vi "ExportMeasuresToHTML.vi"(8 "error in (no error)":errorcluster, 11 "Table in":refnum<vi>) -> (0 "error out":errorcluster)   [LabVIEW 2013]
uses:
  GlobalVariables/UserInfos.vi
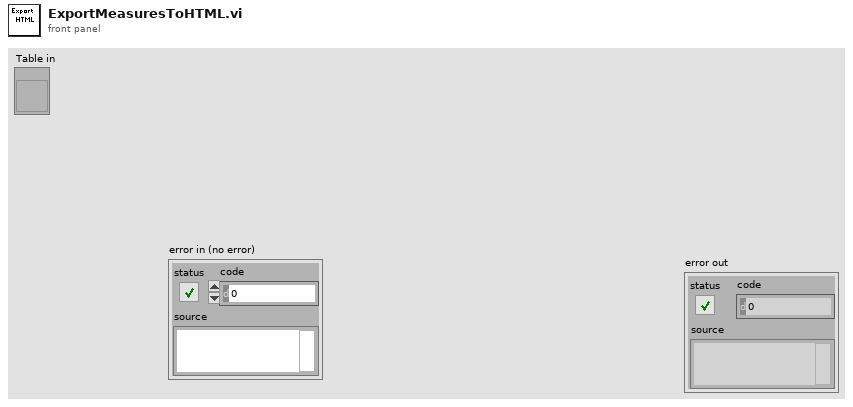
[diagram p1: front panel]
types:
  T1 = enum16{"open", "replace", "create", "open or create", "replace or create", "replace or create with confirmation"}
  T2 = cluster{"location":string, "Field":string, "Company":string, "Lab":string, "Operator":string, "Well":string, "Lat/Long":string, "Formation":string, "Country":string, "Client":string}
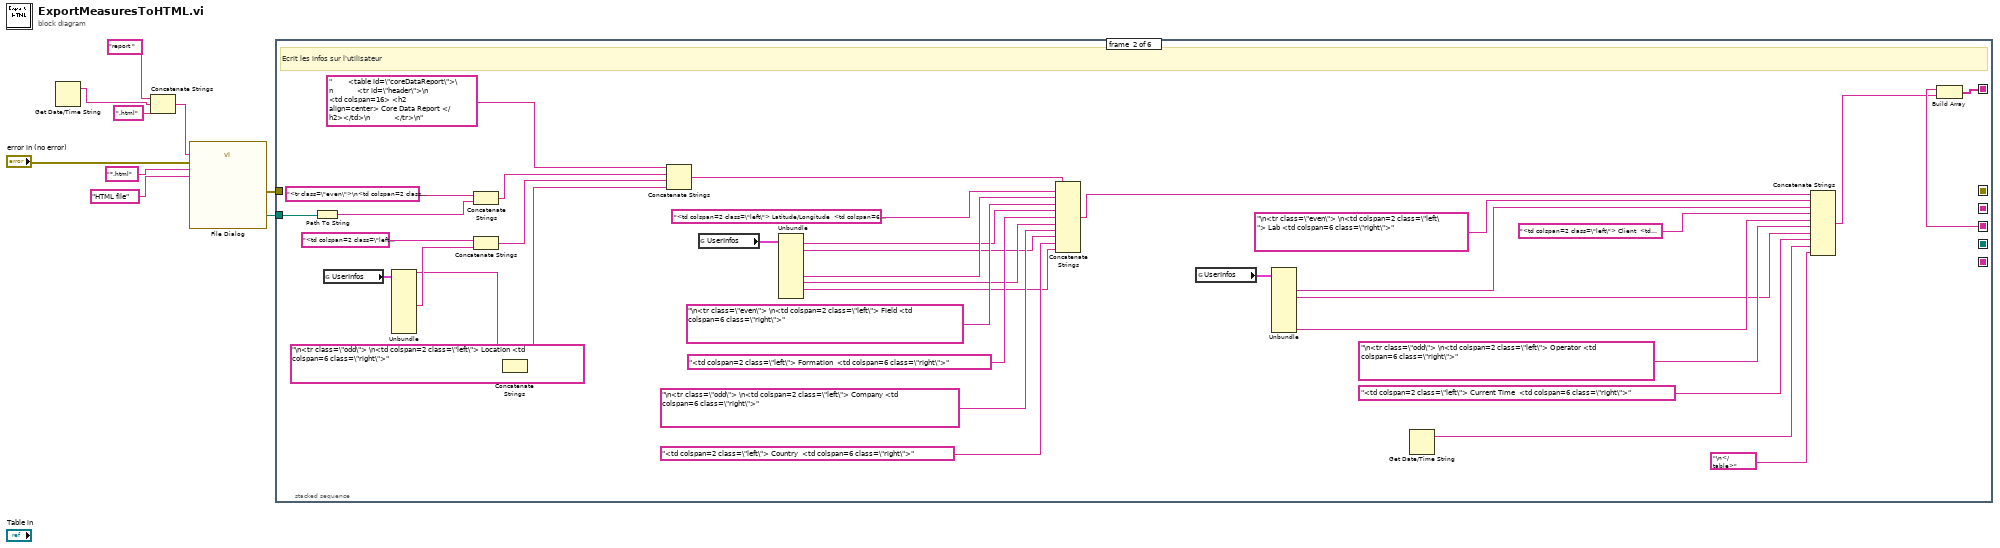
[diagram p0: block diagram]
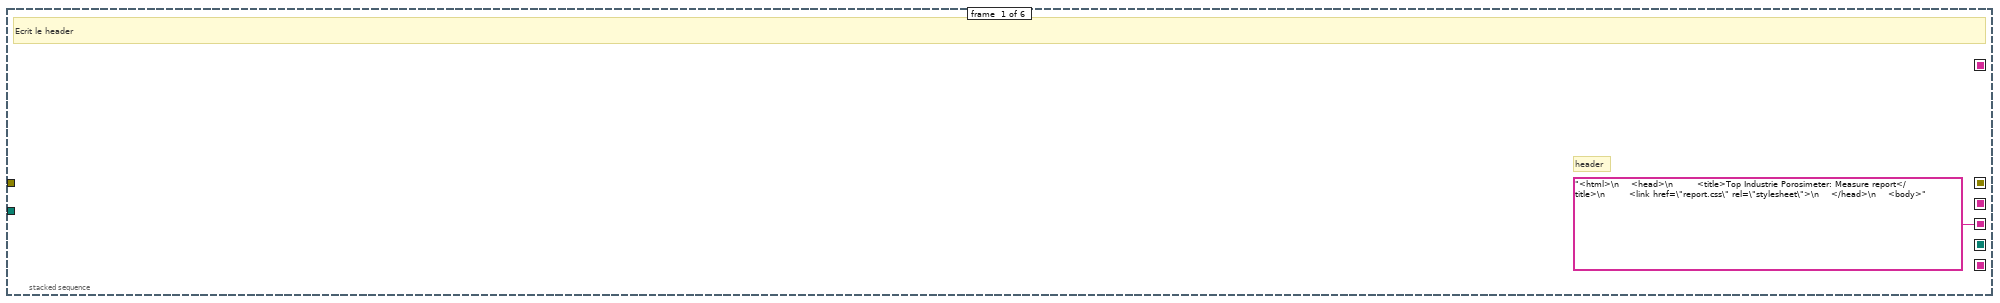
[diagram p2: hidden frame]
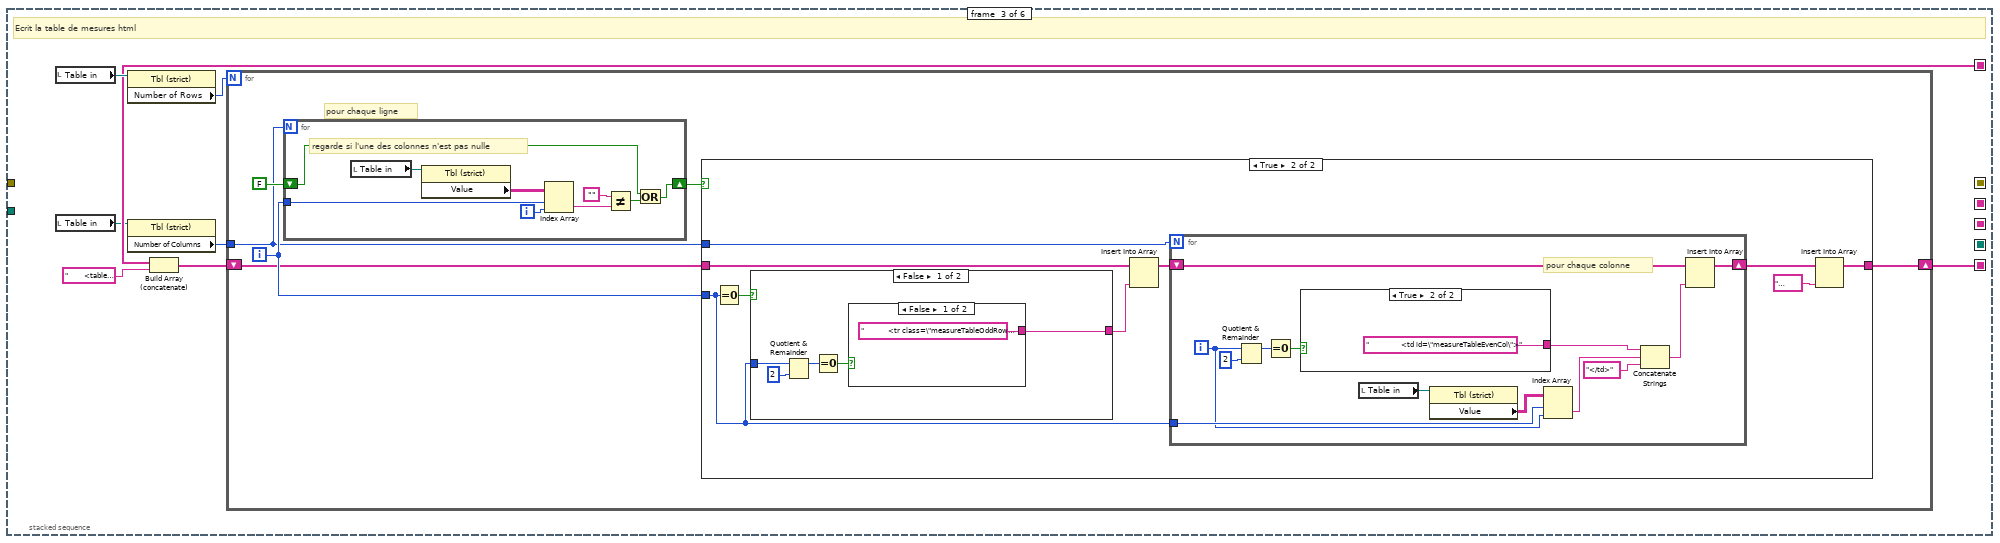
[diagram p3: hidden frame]
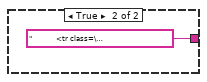
[diagram p5: hidden frame]
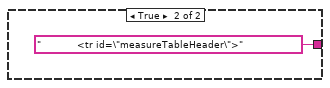
[diagram p6: hidden frame]
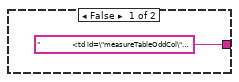
[diagram p7: hidden frame]
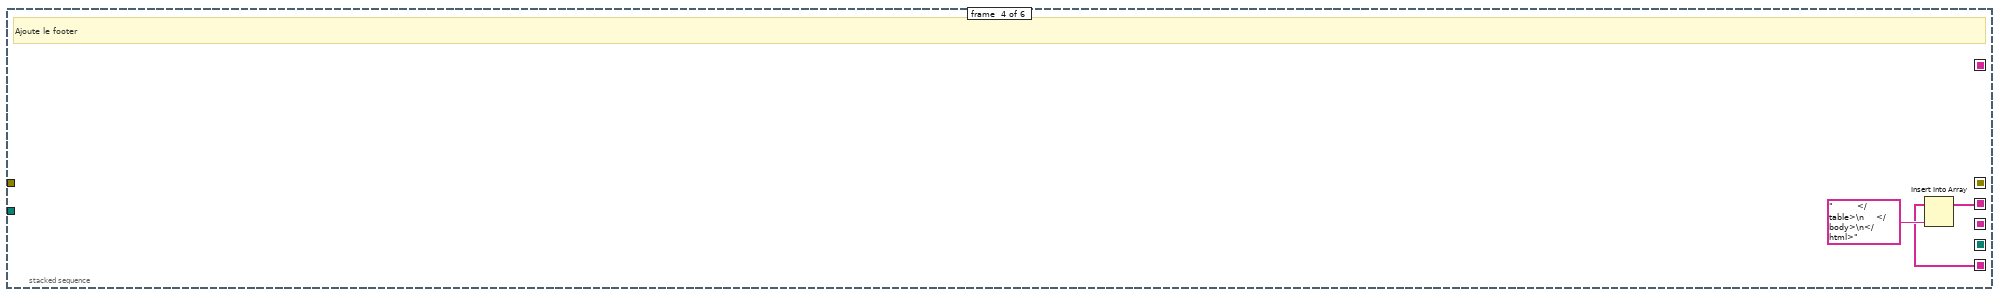
[diagram p8: hidden frame]
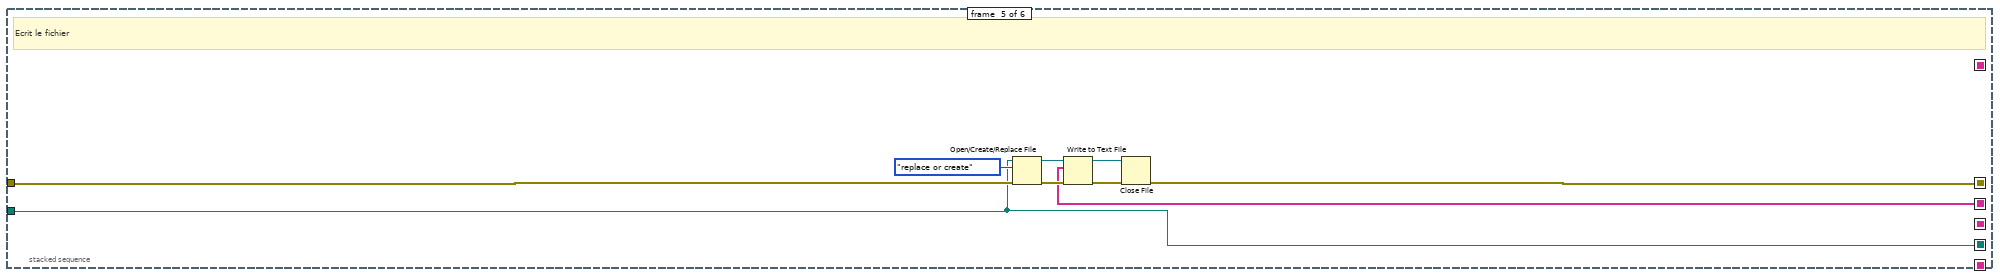
[diagram p9: hidden frame]
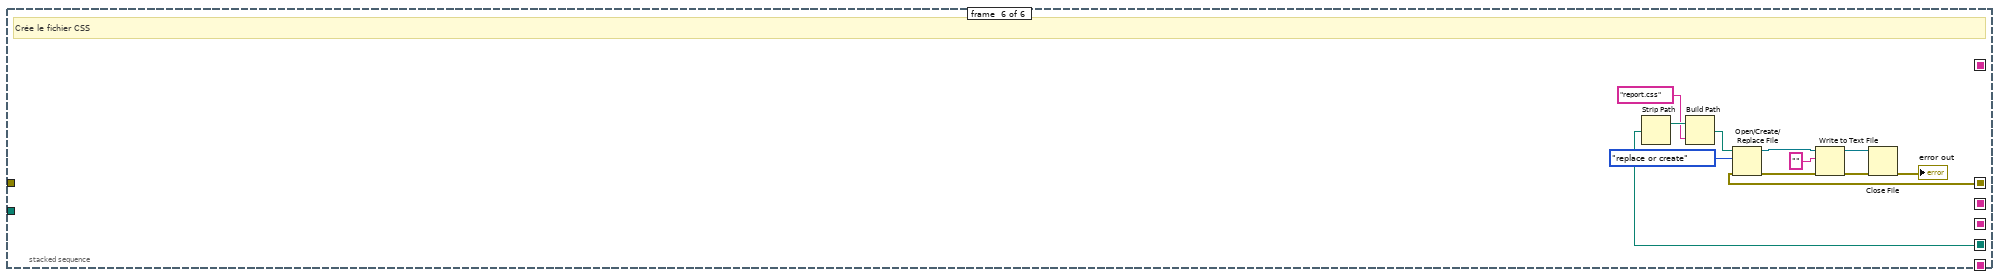
[diagram p10: hidden frame]
diagram:
  n1 = Get Date/Time String() -> (date string=w1:string)  [unwired: 3 in, 1 out]
  n2 = Concatenate Strings("report " ("string"), w1, ".html" ("string")) -> (w2:string)
  n3 = call "File Dialog"("default name"=w2, "error in"="error in (no error)", "pattern (all files)"="*.html", "pattern label"="HTML file") -> ("selected path"=w5:path, "error out"=w6:errorcluster)  [unwired: 8 in, 2 out]
  n4 = stacked-sequence {
    seq-local: ["<html>\n    <head>\n        <title>Top Industrie Porosimeter: Measure report</title>\n        <link href=\"report.css\" rel=\"stylesheet\">\n    </head>\n    <body>" _ _ _ _ _] -> [_ w48 _ _ _ _]
    seq-local: [_ w47 _ _ _ _] -> [_ _ w52 _ _ _]
    seq-local: [_ _ w51 _ _ _] -> [_ _ _ w106 _ _]
    seq-local: [_ _ _ w105 _ _] -> [_ _ _ _ w113 _]
    seq-local: [_ _ _ _ w114 _] -> [_ _ _ _ _ w121]
    seq-local: [_ _ _ _ w108 _] -> [_ _ _ _ _ w117]
    tunnel: w6 -> [_ _ _ _ w109 _]
    tunnel: w5 -> [_ w45 _ _ w108 _]
    frame #0 {
      # "header"
      # "Ecrit le header"
    }
    frame #1 {
      # "Ecrit les infos sur l'utilisateur"
      n5 = Path To String(path=w45) -> (string=w18:string)
      n6 = global read "UserInfos.vi" "UserInfos"() -> (w46:T2)
      n7 = Unbundle(w46) -> ("location"=w14:string, "Well"=w16:string)  [unwired: 8 out]
      n8 = Concatenate Strings("<tr class=\"even\">\n<td colspan=2 class=\"left\"> File Name<td colspan=6 class=\"right\">", w18) -> (w13:string)
      n9 = Concatenate Strings("<td colspan=2 class=\"left\"> Well <td colspan=6 class=\"right\">", w16) -> (w12:string)
      n10 = Concatenate Strings("\n<tr class=\"odd\"> \n<td colspan=2 class=\"left\"> Location <td colspan=6 class=\"right\">", w14) -> (w11:string)
      n11 = Concatenate Strings("        <table id=\"coreDataReport\">\n            <tr id=\"header\">\n                <td colspan=16> <h2 align=center> Core Data Report </h2></td>\n            </tr>\n", w13, w12, w11) -> (w43:string)
      n12 = global read "UserInfos.vi" "UserInfos"() -> (w41:T2)
      n13 = Unbundle(w41) -> ("Field"=w38:string, "Company"=w34:string, "Lat/Long"=w40:string, "Formation"=w36:string, "Country"=w32:string)  [unwired: 5 out]
      n14 = Concatenate Strings(w43, "<td colspan=2 class=\"left\"> Latitude/Longitude  <td colspan=6 class=\"right\">", w40, "\n<tr class=\"even\"> \n<td colspan=2 class=\"left\"> Field <td colspan=6 class=\"right\">", w38, "<td colspan=2 class=\"left\"> Formation  <td colspan=6 class=\"right\">", w36, "\n<tr class=\"odd\"> \n<td colspan=2 class=\"left\"> Company <td colspan=6 class=\"right\">", w34, "<td colspan=2 class=\"left\"> Country  <td colspan=6 class=\"right\">", w32) -> (w31:string)
      n15 = global read "UserInfos.vi" "UserInfos"() -> (w30:T2)
      n16 = Unbundle(w30) -> ("Lab"=w28:string, "Operator"=w24:string, "Client"=w26:string)  [unwired: 7 out]
      n17 = Get Date/Time String() -> (date string=w22:string)  [unwired: 3 in, 1 out]
      n18 = Concatenate Strings(w31, "\n<tr class=\"even\"> \n<td colspan=2 class=\"left\"> Lab <td colspan=6 class=\"right\">", w28, "<td colspan=2 class=\"left\"> Client  <td colspan=6 class=\"right\">", w26, "\n<tr class=\"odd\"> \n<td colspan=2 class=\"left\"> Operator <td colspan=6 class=\"right\">", w24, "<td colspan=2 class=\"left\"> Current Time  <td colspan=6 class=\"right\">", w22, "\n</table>" ("string")) -> (w20:string)
      n19 = Build Array(w48, w20) -> (w47:string[])
    }
    frame #2 {
      # "Ecrit la table de mesures html"
      n20 = local read "Table in"() -> (w55:refnum<vi>)
      n21 = local read "Table in"() -> (w50:refnum<vi>)
      n22 = property on="Property Node" class="Tbl (strict)"(reference=w55) -> ("Number of Rows"=w56:u32)  [unwired: 1 in, 2 out]
      n23 = property on="Property Node" class="Tbl (strict)"(reference=w50) -> ("Number of Columns"=w49:u32)  [unwired: 1 in, 2 out]
      n24 = Build Array (concatenate)(w52, "        <table id=\"measureTable\" >") -> (w54:string[])
      n25 = for {
        N: w56 -> [_]
        shift-right: [w59] -> w51
        shift-left: w54 -> [w58]
        tunnel: w49 -> [w57]
        i -> [w61]
        # "pour chaque ligne"
        n26 = for {
          N: w57 -> [_]
          shift-right: [w71] -> w60
          shift-left: FALSE -> [w70]
          tunnel: w61 -> [w68]
          i -> [w67]
          # "regarde si l'une des colonnes n'est pas nulle"
          n27 = local read "Table in"() -> (w63:refnum<vi>)
          n28 = property on="Property Node" class="Tbl (strict)"(reference=w63) -> ("Value"=w69:string[][])  [unwired: 1 in, 2 out]
          n29 = Index Array(array=w69, index (row)=w68, index (col)=w67) -> (element=w66:string)
          n30 = Not Equal?(x="", y=w66) -> (x != y?=w64:bool)
          n31 = Or(x=w70, y=w64) -> (x .or. y?=w71:bool)
        }
        n32 = case shown="True" w60 {
          tunnel: w57 -> [_ w81]
          tunnel: w58 -> [w72 w78]
          tunnel: w61 -> [_ w75]
          tunnel: [w72 w80] -> w59
          frame False {
          }
          frame True {
            n33 = Equal To 0?(x=w75) -> (x = 0?=w77:bool)
            n34 = case shown="False" w77 {
              tunnel: [w86 "            <tr id=\"measureTableHeader\">"] -> w73
              tunnel: w75 -> [w82 _]
              frame False {
                n35 = Quotient & Remainder(x=w82, y=2) -> (x-y*floor(x/y)=w83:i32)  [unwired: 1 out]
                n36 = Equal To 0?(x=w83) -> (x = 0?=w84:bool)
                n37 = case shown="False" w84 {
                  tunnel: ["            <tr class=\"measureTableOddRow\">" "            <tr class=\"measureTableEvenRow\">"] -> w86
                  frame False {
                  }
                  frame True {
                  }
                }
              }
              frame True {
              }
            }
            n38 = Insert Into Array(array=w78, new element=w73) -> (w76:string[])  [unwired: 1 in]
            n39 = for {
              N: w81 -> [_]
              shift-right: [w101] -> w79
              shift-left: w76 -> [w102]
              tunnel: w75 -> [w99]
              i -> [w94]
              # "pour chaque colonne"
              n40 = Quotient & Remainder(x=w94, y=2) -> (x-y*floor(x/y)=w96:i32)  [unwired: 1 out]
              n41 = Equal To 0?(x=w96) -> (x = 0?=w93:bool)
              n42 = case shown="True" w93 {
                tunnel: ["                <td id=\"measureTableOddCol\" >" "                <td id=\"measureTableEvenCol\">"] -> w90
                frame False {
                }
                frame True {
                }
              }
              n43 = local read "Table in"() -> (w97:refnum<vi>)
              n44 = property on="Property Node" class="Tbl (strict)"(reference=w97) -> ("Value"=w100:string[][])  [unwired: 1 in, 2 out]
              n45 = Index Array(array=w100, index (row)=w99, index (col)=w94) -> (element=w98:string)
              n46 = Concatenate Strings(w90, w98, "</td>") -> (w91:string)
              n47 = Insert Into Array(array=w102, new element=w91) -> (w101:string[])  [unwired: 1 in]
            }
            n48 = Insert Into Array(array=w79, new element="            </tr>") -> (w80:string[])  [unwired: 1 in]
          }
        }
      }
    }
    frame #3 {
      # "Ajoute le footer"
      n49 = Insert Into Array(array=w106, new element="        </table>\n    </body>\n</html>") -> (w105:string[])  [unwired: 1 in]
    }
    frame #4 {
      # "Ecrit le fichier"
      n50 = Open/Create/Replace File(file path (use dialog)=w108, error in=w109, operation (0:open)=T1."replace or create") -> (refnum out=w112:refnum<file>, error out=w115:errorcluster)  [unwired: 3 in, 1 out]
      n51 = Write to Text File(file (use dialog)=w112, text=w113, error in=w115) -> (refnum out=w110:refnum<file>, error out=w116:errorcluster)  [unwired: 1 in, 1 out]
      n52 = Close File(refnum=w110, error in=w116) -> (error out=w114:errorcluster)  [unwired: 1 out]
    }
    frame #5 {
      # "Crée le fichier CSS"
      n53 = Strip Path(path=w117) -> (stripped path=w120:path)  [unwired: 1 out]
      n54 = Build Path(base path=w120, name or relative path="report.css") -> (appended path=w118:path)
      n55 = Open/Create/Replace File(file path (use dialog)=w118, error in=w121, operation (0:open)=T1."replace or create") -> (refnum out=w126:refnum<file>, error out=w124:errorcluster)  [unwired: 3 in, 1 out]
      n56 = Write to Text File(file (use dialog)=w126, text="", error in=w124) -> (refnum out=w127:refnum<file>, error out=w125:errorcluster)  [unwired: 1 in, 1 out]
      n57 = Close File(refnum=w127, error in=w125) -> (error out=→"error out":errorcluster)  [unwired: 1 out]
    }
  }
